vi "AlliGator 2-Exp Decay Model.vi"(9 "Fit Simulation Parameters":T2, 10 "Period":dbl[unit], 11 "Decay Simulation Parameters":T1) -> (3 "Output Plot":cluster{"t Array":dbl[], "I Array":dbl[]})   [LabVIEW 2021, in "AlliGator Fit Method Benchmark.lvlib"]
doc: "Computes a 2-#xp decay with the provided parameters."
uses:
  AlliGator Fit Method Benchmark.lvlib
  AlliGator Fit Simulation Parameters.ctl
  AlliGator Decay Simulation Parameters.ctl
  a57d32fc-67bf-49bc-8847-bf20d45ab2ab.vi
panel:
  # "see the AlliGator License on the block diagram (Ctrl+E or Window:Show Block Diagram)"
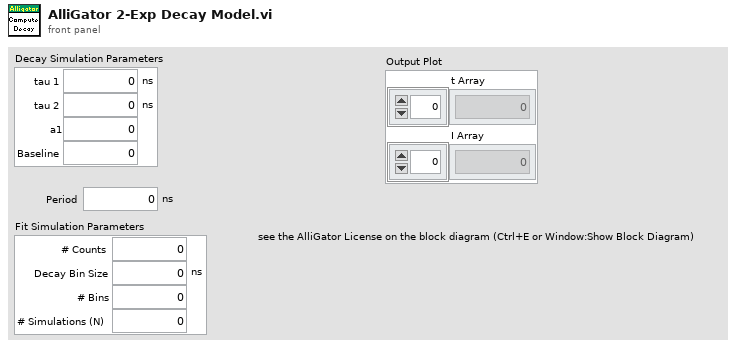
[diagram p1: front panel]
types:
  T1 = typedef "AlliGator Fit Method Benchmark.lvlib/AlliGator Decay Simulation Parameters.ctl" = cluster{"tau 1":dbl[unit], "tau 2":dbl[unit], "a1":dbl, "Baseline":dbl}
  T2 = typedef "AlliGator Fit Method Benchmark.lvlib/AlliGator Fit Simulation Parameters.ctl" = cluster{"# Counts":i32, "# Simulations (N)":i32, "Decay Bin Size":dbl[unit], "# Bins":i32}
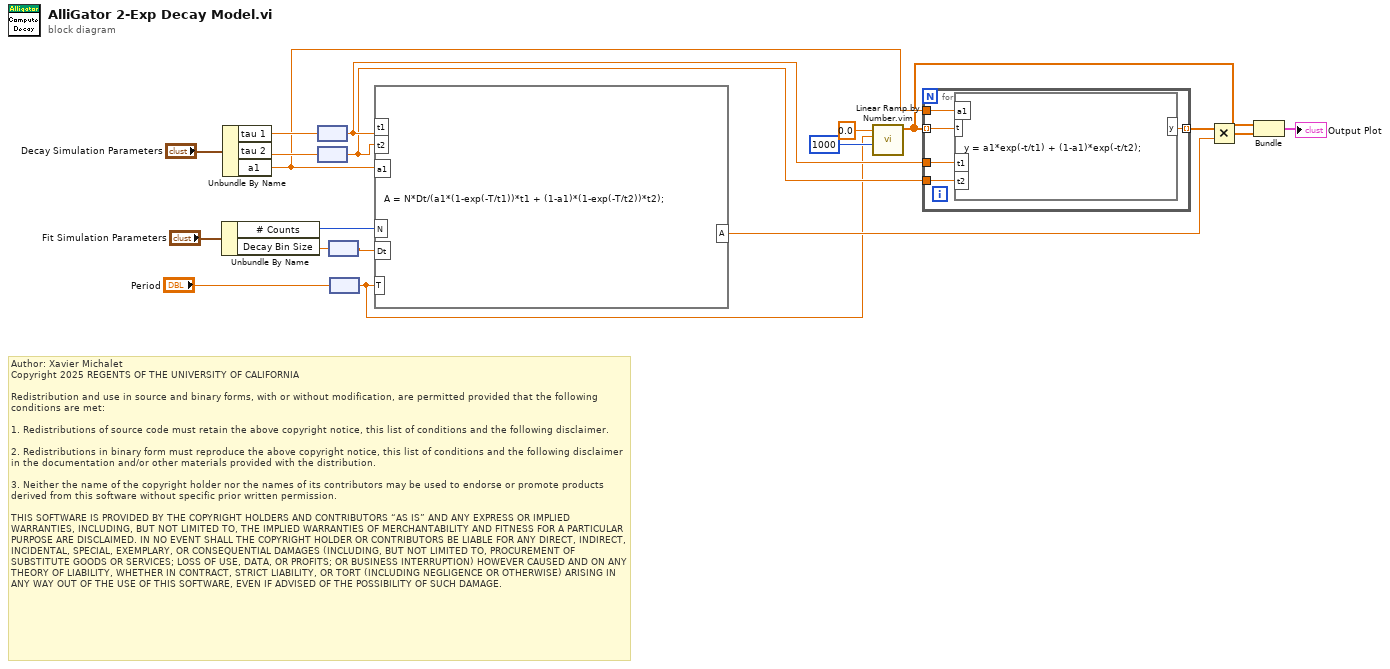
[diagram p0: block diagram]
diagram:
  # "Author: Xavier Michalet\nCopyright 2025 REGENTS OF THE UNIVERSITY OF CALIFORNIA\n\nRedistribution and use in source and binary forms, with or without modification, are permitted provided that the following conditions are met:\n\n1. Redistributions of source code must retain the above copyright notice, this list of conditions and the following disclaimer.\n\n2. Redistributions in binary form must reproduce the above copyright notice, this list of conditions and the following disclaimer in the documentation and/or other materials provided with the distribution.\n\n3. Neither the name of the copyright holder nor the names of its contributors may be used to endorse or promote products derived from this software without specific prior written permission.\n\nTHIS SOFTWARE IS PROVIDED BY THE COPYRIGHT HOLDERS AND CONTRIBUTORS “AS IS” AND ANY EXPRESS OR IMPLIED WARRANTIES, INCLUDING, BUT NOT LIMITED TO, THE IMPLIED WARRANTIES OF MERCHANTABILITY AND FITNESS FOR A PARTICULAR PURPOSE ARE DISCLAIMED. IN NO EVENT SHALL THE COPYRIGHT HOLDER OR CONTRIBUTORS BE LIABLE FOR ANY DIRECT, INDIRECT, INCIDENTAL, SPECIAL, EXEMPLARY, OR CONSEQUENTIAL DAMAGES (INCLUDING, BUT NOT LIMITED TO, PROCUREMENT OF SUBSTITUTE GOODS OR SERVICES; LOSS OF USE, DATA, OR PROFITS; OR BUSINESS INTERRUPTION) HOWEVER CAUSED AND ON ANY THEORY OF LIABILITY, WHETHER IN CONTRACT, STRICT LIABILITY, OR TORT (INCLUDING NEGLIGENCE OR OTHERWISE) ARISING IN ANY WAY OUT OF THE USE OF THIS SOFTWARE, EVEN IF ADVISED OF THE POSSIBILITY OF SUCH DAMAGE."
  n1 = Unbundle By Name("Fit Simulation Parameters") -> ("# Counts"=w15:i32, "Decay Bin Size"=w14:dbl[unit])
  n2 = Unbundle By Name("Decay Simulation Parameters") -> ("tau 1"=w17:dbl[unit], "tau 2"=w16:dbl[unit], "a1"=w10:dbl)
  n3 = node(w17) -> (w9:dbl)
  n4 = node(w16) -> (w8:dbl)
  n5 = node(w14) -> (w1:dbl)
  n6 = node("Period") -> (w2:dbl)
  n7 = formula code="A = N*Dt/(a1*(1-exp(-T/t1))*t1 + (1-a1)*(1-exp(-T/t2))*t2);"("t1"=w9, "t2"=w8, "a1"=w10, "N"=w15, "Dt"=w1, "T"=w2) -> ("A"=w6:dbl)
  n8 = call "Linear Ramp by Number.vim"("# Steps (1)"=1000 ("# Elements (1)"), "End (1)"=w2, "Start (0)"=0.0) -> ("Ramp"=w4:dbl[])  [unwired: 6 in, 2 out]
  n9 = for {
    tunnel: w4 -> [w24] mode=indexing
    tunnel: w10 -> [w23]
    tunnel: w9 -> [w22]
    tunnel: w8 -> [w21]
    tunnel: [w20] -> w7 mode=indexing
    n10 = formula code="y = a1*exp(-t/t1) + (1-a1)*exp(-t/t2);"("t"=w24, "a1"=w23, "t1"=w22, "t2"=w21) -> ("y"=w20:dbl)
  }
  n11 = Multiply(x=w7, y=w6) -> (x*y=w5:dbl[])
  n12 = Bundle("Ramp"=w4, w5) -> (→"Output Plot":cluster{"Ramp":dbl[], dbl[]})  [unwired: 1 in]
